vi "短信语音配置.vi"(10 "电话":string, 11 "姓名":string) -> (1 "输出":bool, 2 "电话输出":string, 3 "姓名输出":string)   [LabVIEW 2016, in "Alarm interface.lvlib" / "短信语音库.lvlib"]
panel:
  in  "取消":bool
  in  "确定":bool
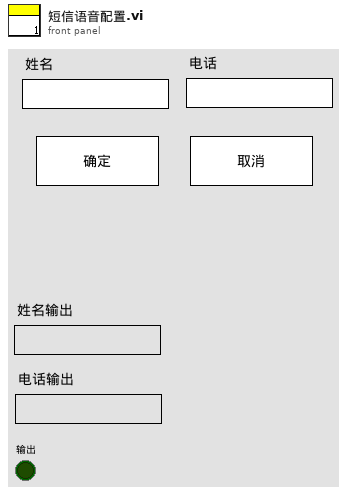
[diagram p1: front panel]
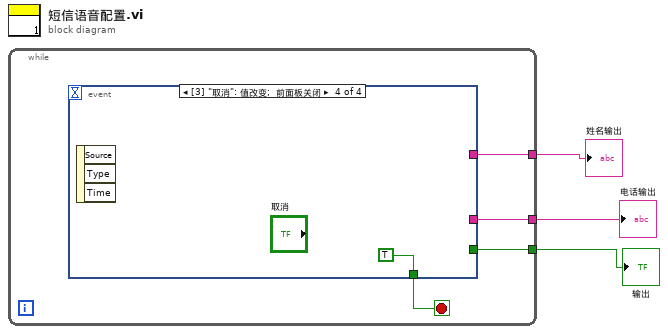
[diagram p0: block diagram]
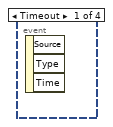
[diagram p2: hidden frame]
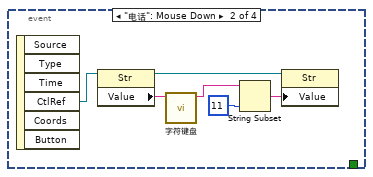
[diagram p3: hidden frame]
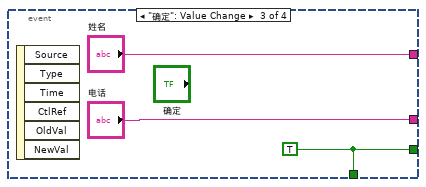
[diagram p4: hidden frame]
diagram:
  n1 = while {
    tunnel: [w7] -> w3
    tunnel: [w6] -> w2
    tunnel: [w5] -> w1
    stop <- w4 stop-if-true
    n2 = event shown="[3] \"取消\": 值改变;  前面板关闭" {
      selector: _ -> [_ _ _ _]
      dyn-events: _ -> [_ _ _ _]
      timeout: _ -> [_ _ _ _]
      tunnel: [_ _ "姓名" _] -> w7
      tunnel: [_ _ "电话" _] -> w6
      tunnel: [_ _ w14 _] -> w5
      tunnel: [_ _ w14 TRUE] -> w4
      event Timeout {
        n3 = event-data() -> ()  [unwired: 1 in, 3 out]
      }
      event "电话": Mouse Down {
        n4 = event-data() -> ("CtlRef"=w8:refnum<vi>)  [unwired: 1 in, 5 out]
        n5 = property class="Str"(reference=w8) -> (reference out=w11:refnum<vi>, "Value"=w13:string)  [unwired: 1 in, 1 out]
        n6 = call "字符键盘.vi"("Old String"=w13) -> ("String"=w12:string)  [unwired: 10 in]
        n7 = String Subset(string=w12, length (rest)=11 ("长度（剩余）")) -> (substring=w10:string)  [unwired: 1 in]
        n8 = property class="Str"(reference=w11, "Value"=w10) -> ()  [unwired: 1 in, 2 out]
      }
      event "确定": Value Change {
        w14 = TRUE
        n9 = event-data() -> ()  [unwired: 1 in, 6 out]
      }
      event "取消": Value Change; Panel Close {
        n10 = event-data() -> ()  [unwired: 1 in, 3 out]
      }
    }
  }
  "姓名输出" <- w3
  "电话输出" <- w2
  "输出" <- w1
